vi "Get Range Utilization.vi"(0 "waveforms in":waveform(dbl)[](array[waveform]), 5 "full-range RMS values":dbl[](array[numeric]), 9 "system info in":refnum<class "EP System Info.lvclass">, 11 "error in (no error)":errorcluster) -> (4 "waveforms out":waveform(dbl)[](array[waveform]), 10 "system info out":refnum<class "EP System Info.lvclass">, 14 "actual ranges [%]":dbl[](array[numeric]), 15 "error out":errorcluster)   [LabVIEW 2014, in "NI_EP_Power Quality.lvlib"]
doc: "Calculates the range utilization, in percentage, of voltage waveforms, current waveforms, or waveforms that contain both voltage and current. Range utilization is the ratio of the actual RMS value to the nominal RMS value of the voltage or current.\n\nThis VI supports measuring single-line and multiple-line systems."
uses:
  <vilib>/addons/Electrical Power/PQ/NI_EP_Power Quality.lvlib
  <vilib>/addons/Electrical Power/PQ/Common/Classes/System Info/EP System Info.lvclass
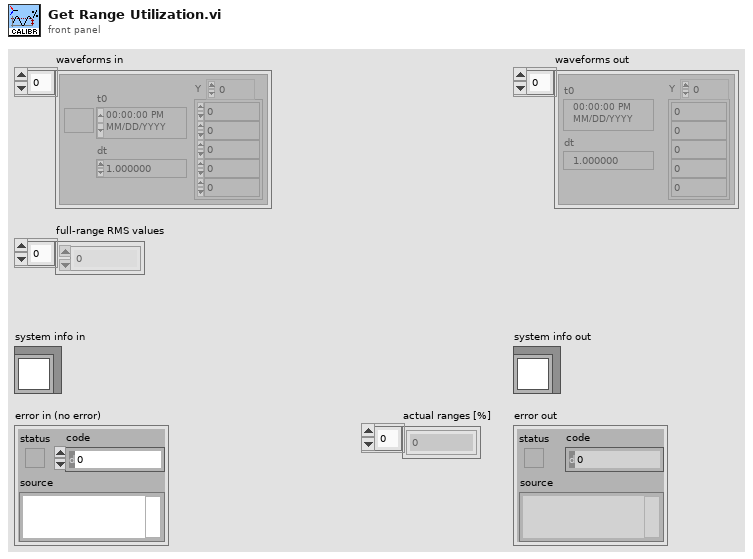
[diagram p1: front panel]
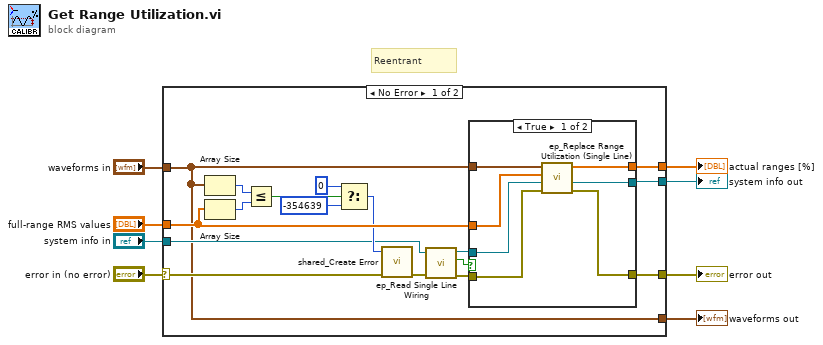
[diagram p0: block diagram]
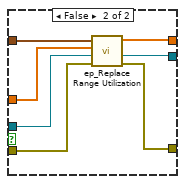
[diagram p2: hidden frame]
diagram:
  # "Reentrant"
  n1 = case shown="No Error" "error in (no error)" {
    selector: "error in (no error)" -> [w10 w42]
    tunnel: [w25 _] -> w8
    tunnel: "full-range RMS values" -> [w22 _]
    tunnel: [w20 w41] -> w6
    tunnel: "waveforms in" -> [w9 w40]
    tunnel: [w19 w42] -> w4
    tunnel: "system info in" -> [w15 w41]
    tunnel: [w9 w40] -> w1
    frame No Error {
      n2 = Array Size(array=w9) -> (size(s)=w23:i32)
      n3 = Array Size(array=w22) -> (size(s)=w24:i32)
      n4 = Less Or Equal?(x=w23, y=w24) -> (x <= y?=w21:bool)
      n5 = Select(t=0 ("error code (0)"), s=w21, f=-354639 ("error code (0)")) -> (s? t:f=w16:i32)
      n6 = call <vilib>:"shared_Create Error.vi"("error in (no error)"=w10, "error code (0)"=w16) -> ("error out"=w13:errorcluster)  [unwired: 9 in]
      n7 = call <vilib>:"ep_Read Single Line Wiring.vi"("error in (no error)"=w13, "system info in"=w15) -> ("error out"=w12:errorcluster, "single line wiring? (F)"=w11:bool, "system info out"=w14:refnum<class "EP System Info.lvclass">)  [unwired: 7 in]
      n8 = case shown="True" w11 {
        tunnel: [w28 w33] -> w25
        tunnel: w22 -> [w31 w38]
        tunnel: [w27 w35] -> w20
        tunnel: w9 -> [w32 w39]
        tunnel: [w26 w34] -> w19
        tunnel: w14 -> [w30 w37]
        tunnel: w12 -> [w29 w36]
        frame True {
          n9 = call <vilib>:"ep_Replace Range Utilization (Single Line).vi"("error in (no error)"=w29, "system info in"=w30, "full-range RMS values"=w31, "waveforms in"=w32) -> ("error out"=w26:errorcluster, "system info out"=w27:refnum<class "EP System Info.lvclass">, "actual ranges [%]"=w28:dbl[])  [unwired: 5 in]
        }
        frame False {
          n10 = call <vilib>:"ep_Replace Range Utilization.vi"("error in (no error)"=w36, "system info in"=w37, "full-range RMS values"=w38, "waveforms in"=w39) -> ("error out"=w34:errorcluster, "system info out"=w35:refnum<class "EP System Info.lvclass">, "actual ranges [%]"=w33:dbl[])  [unwired: 5 in]
        }
      }
    }
    frame Error {
    }
  }
  "error out" <- w4
  "actual ranges [%]" <- w8
  "system info out" <- w6
  "waveforms out" <- w1
